vi "Task Uninit.vi"(8 "error in (no error)":errorcluster, 11 "DaqAnalogIn in":refnum<class "DaqAnalogIn.lvclass">) -> (0 "error out":errorcluster, 3 "DaqAnalogIn out":refnum<class "DaqAnalogIn.lvclass">)   [LabVIEW 2020, in "VolatusDaq.lvlib" / "DaqAnalogIn.lvclass"]
uses:
  DaqAnalogIn.lvclass
  DaqAnalogIn.lvclass/DaqAnalogIn.ctl
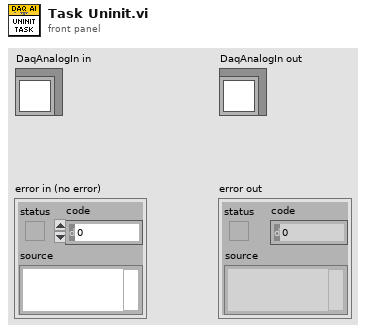
[diagram p1: front panel]
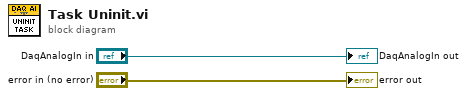
[diagram p0: block diagram]
diagram:
  "error out" <- "error in (no error)"
  "DaqAnalogIn out" <- "DaqAnalogIn in"
